vi "Activation - License Info.vi"(8 "Error In":errorcluster, 11 "License Param":T1) -> (0 "Error Out":errorcluster, 3 "License Info":string)   [LabVIEW 2020]
uses:
  Control/License File Parameter.ctl
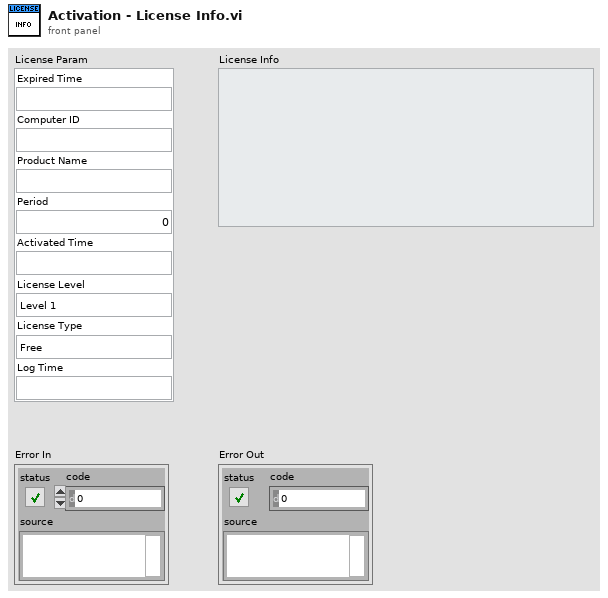
[diagram p1: front panel]
types:
  T1 = typedef "License File Parameter.ctl" = cluster{"Expired Time":string, "Computer ID":string, "Product Name":string, "Period":i16, "Activated Time":string, "License Level":enum16{"Level 1", "Level 2", "Level 3", "Level 4", "Level 5"}, "License Type":enum16{"Free", "Trial", "Subscription", "Perpetual"}, "Log Time":string}
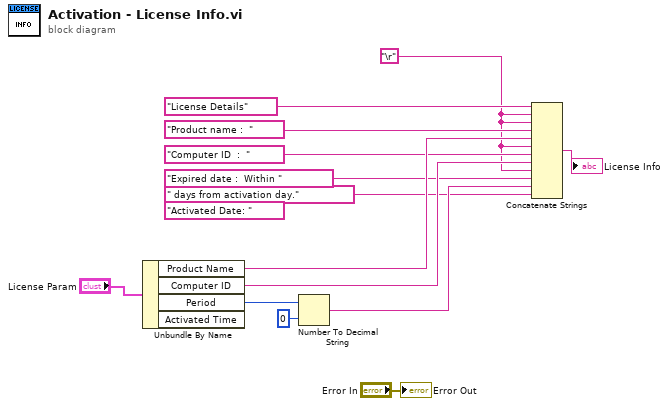
[diagram p0: block diagram]
diagram:
  (unwired) "Activated Date: "
  w1 = "\r"
  n1 = Unbundle By Name("License Param") -> ("Product Name"=w11:string, "Computer ID"=w9:string, "Period"=w6:i16)  [unwired: 1 out]
  n2 = Number To Decimal String(number=w6, width (-)=i16 0) -> (decimal integer string=w5:string)
  n3 = Concatenate Strings("License Details", w1, w1, "Product name :  ", w11, w1, "Computer ID  :  ", w9, w1, "Expired date :  Within ", w5, " days from activation day.") -> (→"License Info":string)
  "Error Out" <- "Error In"
